vi "QuickFWCopy.vi"(8 "Error In":errorcluster, 10 "Override lib path?":bool, 11 "Arduino lib directory":path) -> (0 "Error Out":errorcluster)   [LabVIEW 2019, in "LINXx.lvlib"]
uses:
  LINXx.lvlib
  <vilib>/MakerHub/LINX/Private/Type Defs/Firmware Library Component.ctl
  <vilib>/Utility/config.llb/Read Key (String).vi
  <vilib>/Utility/config.llb/NI_LVConfig.lvlib
  <vilib>/MakerHub/Toolbox/LMH-Toolbox.lvlib
  <vilib>/MakerHub/LINX/LMH-LINX.lvlib
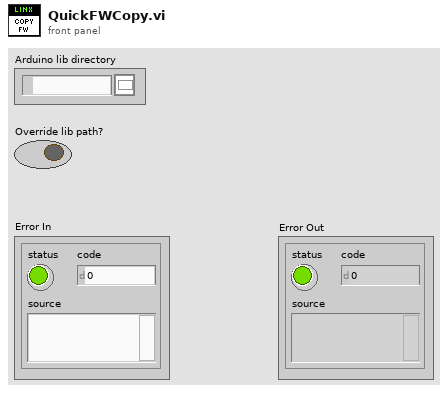
[diagram p1: front panel]
types:
  T1 = typedef "NI_LVConfig.lvlib/Config Data RefNum.ctl" = refnum<k1>
  T2 = typedef "LMH-LINX.lvlib/Firmware Library Component.ctl" = cluster{"Source":path, "Destination":path}
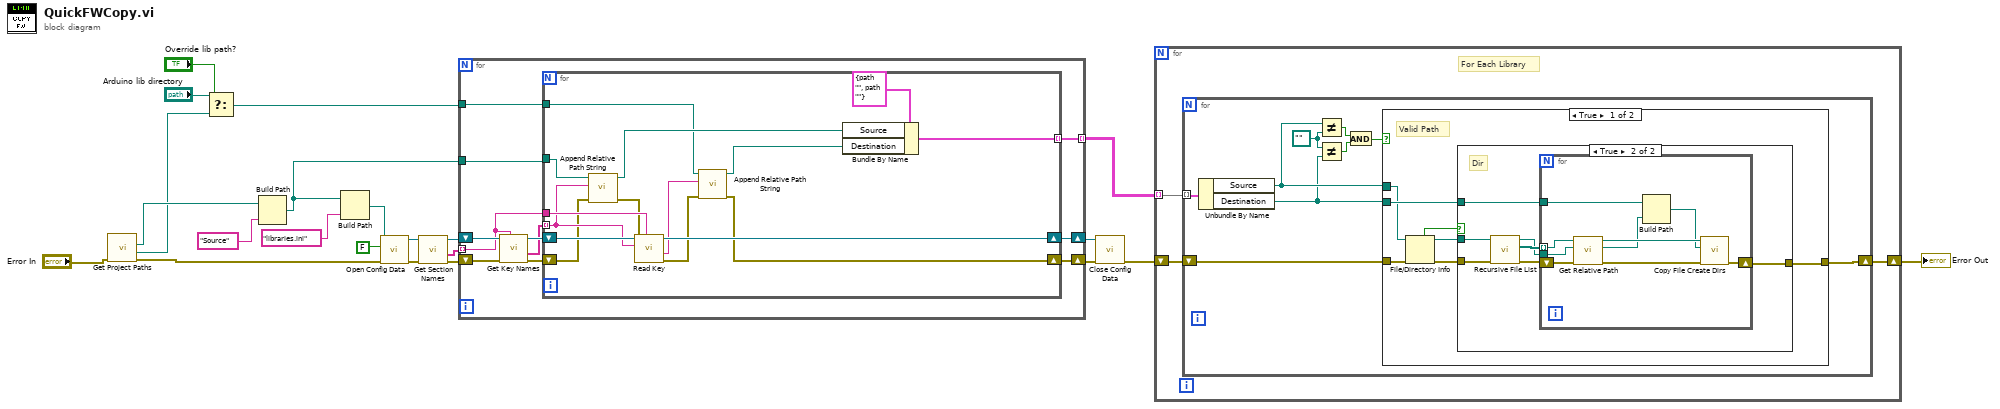
[diagram p0: block diagram]
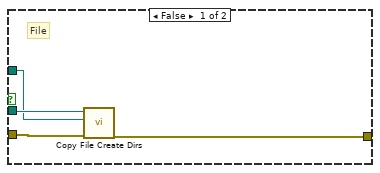
[diagram p2: hidden frame]
diagram:
  n1 = call "Get Project Paths.vi"("error in (no error)"="Error In") -> ("error out"=w6:errorcluster, "PlatformIO lib path"=w3:path, "Firmware path"=w5:path)  [unwired: 7 in, 1 out]
  n2 = Select(t="Arduino lib directory", s="Override lib path?", f=w3) -> (s? t:f=w4:path)
  n3 = Build Path(base path=w5, name or relative path="Source") -> (appended path=w8:path)
  n4 = Build Path(base path=w8, name or relative path="libraries.ini") -> (appended path=w11:path)
  n5 = call <vilib>:"Open Config Data.vi"("error in (no error)"=w6, "create file if necessary (T)"=FALSE, "configuration file path"=w11) -> ("error out"=w21:errorcluster, "refnum"=w22:T1)  [unwired: 6 in, 1 out]
  n6 = call <vilib>:"Get Section Names.vi"("error in (no error)"=w21, "refnum"=w22) -> ("error out"=w17:errorcluster, "section names"=w15:string[], "refnum out"=w19:T1)  [unwired: 7 in]
  n7 = for {
    shift-right: [w30] -> w18
    shift-left: w19 -> [w33]
    shift-right: [w28] -> w16
    shift-left: w17 -> [w32]
    tunnel: w15 -> [w26] mode=indexing
    tunnel: w8 -> [w25]
    tunnel: [w24] -> w14 mode=indexing
    tunnel: w4 -> [w23]
    n8 = call <vilib>:"Get Key Names.vi"("section"=w26, "error in (no error)"=w32, "refnum"=w33) -> ("error out"=w29:errorcluster, "key names"=w27:string[], "refnum out"=w31:T1)  [unwired: 5 in, 1 out]
    n9 = for {
      shift-right: [w47] -> w30
      shift-left: w31 -> [w48]
      shift-right: [w38] -> w28
      shift-left: w29 -> [w40]
      tunnel: w27 -> [w41] mode=indexing
      tunnel: w26 -> [w46]
      tunnel: w25 -> [w42]
      tunnel: [w35] -> w24 mode=indexing
      tunnel: w23 -> [w34]
      n10 = call <vilib>:"Append Relative Path String.vi"("Error In"=w40, "Relative Path"=w41, "Base Path"=w42) -> ("Error Out"=w39:errorcluster, "Absolute Path"=w37:path)  [unwired: 7 in]
      n11 = call-poly <vilib>:"Read Key.vi"("section"=w46, "error in (no error)"=w39, "key"=w41, "refnum"=w48) -> ("error out"=w45:errorcluster, "value"=w44:string, "refnum out"=w47:T1)  [unwired: 4 in, 1 out]
      n12 = call <vilib>:"Append Relative Path String.vi"("Error In"=w45, "Relative Path"=w44, "Base Path"=w34) -> ("Error Out"=w38:errorcluster, "Absolute Path"=w36:path)  [unwired: 7 in]
      n13 = Bundle By Name(cluster=T2 {"Source"=path "", "Destination"=path ""} ("Library Component"), "Source"=w37, "Destination"=w36) -> (w35:T2)
    }
  }
  n14 = call <vilib>:"Close Config Data.vi"("error in (no error)"=w16, "refnum"=w18) -> ("error out"=w13:errorcluster)  [unwired: 8 in, 1 out]
  n15 = for {
    tunnel: w14 -> [w50] mode=indexing
    shift-right: [w49] -> w12
    shift-left: w13 -> [w51]
    # "For Each Library"
    n16 = for {
      tunnel: w50 -> [w60] mode=indexing
      shift-right: [w59] -> w49
      shift-left: w51 -> [w52]
      w56 = path ""
      n17 = Unbundle By Name(w60) -> ("Source"=w55:path, "Destination"=w54:path)
      n18 = Not Equal?(x=w55, y=w56) -> (x != y?=w58:bool)
      n19 = Not Equal?(x=w56, y=w54) -> (x != y?=w57:bool)
      n20 = And(x=w58, y=w57) -> (x .and. y?=w53:bool)
      n21 = case shown="True" w53 {
        tunnel: [w66 w88] -> w59
        tunnel: w54 -> [w67 _]
        tunnel: w55 -> [w64 _]
        tunnel: w52 -> [w65 w88]
        frame True {
          # "Valid Path"
          n22 = File/Directory Info(path=w64, error in=w65) -> (path out=w63:path, directory=w61:bool, error out=w62:errorcluster)  [unwired: 4 out]
          n23 = case shown="True" w61 {
            tunnel: w67 -> [w69 w75]
            tunnel: [w68 w74] -> w66
            tunnel: w63 -> [w70 w73]
            tunnel: w62 -> [w71 w72]
            frame False {
              # "File"
              n24 = call <vilib>:"Copy File Create Dirs.vi"("Error In"=w71, "Destination"=w69, "Source"=w70) -> ("Error Out"=w68:errorcluster)  [unwired: 8 in]
            }
            frame True {
              # "Dir"
              n25 = call <vilib>:"Recursive File List.vi"("error in (no error)"=w72, "Folder Path"=w73) -> ("error out"=w78:errorcluster, "All Files in Dir"=w77:path[], "dup Folder Path"=w76:path)  [unwired: 5 in, 2 out]
              n26 = for {
                tunnel: w77 -> [w86] mode=indexing
                tunnel: w76 -> [w85]
                tunnel: w75 -> [w82]
                shift-right: [w79] -> w74
                shift-left: w78 -> [w87]
                n27 = call <vilib>:"Get Relative Path.vi"("Error In"=w87, "Relative Path Root"=w85, "File / Folder"=w86) -> ("Error Out"=w84:errorcluster, "Relative Path"=w81:path, "Duplicate File / Folder"=w83:path)  [unwired: 6 in]
                n28 = Build Path(base path=w82, name or relative path=w81) -> (appended path=w80:path)
                n29 = call <vilib>:"Copy File Create Dirs.vi"("Error In"=w84, "Destination"=w80, "Source"=w83) -> ("Error Out"=w79:errorcluster)  [unwired: 8 in]
              }
            }
          }
        }
        frame False {
          # "Invalid Path"
        }
      }
    }
  }
  "Error Out" <- w12
